vi "Lockin.DAQ.Generate.Waveforms.vi"(4 "sweep index":i32=-1, 6 "Reset Phase?":bool, 8 "error in (no error)":errorcluster, 11 "Instrument.DAQ":refnum<class "Instrument.DAQ.lvclass">) -> (0 "error out":errorcluster, 3 "Instrument.DAQ":refnum<class "Instrument.DAQ.lvclass">)   [LabVIEW 2019, in "Instrument.DAQ.lvclass"]
uses:
  Instrument.DAQ.lvclass
  Instrument.DAQ.lvclass/Instrument.DAQ.ctl
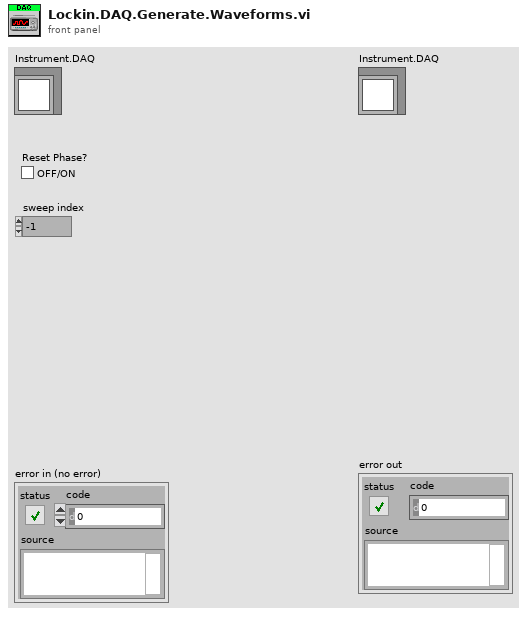
[diagram p1: front panel]
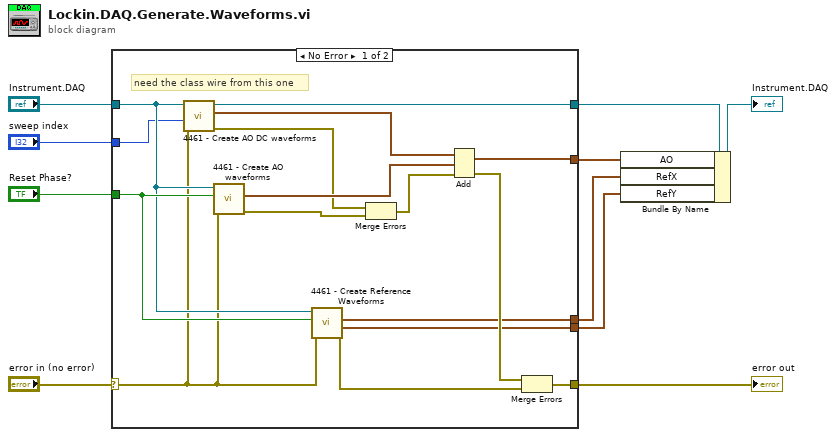
[diagram p0: block diagram]
diagram:
  n1 = case shown="No Error" "error in (no error)" {
    selector: "error in (no error)" -> [w23 w28]
    tunnel: [w11 _] -> w2
    tunnel: "Reset Phase?" -> [w26 _]
    tunnel: [w18 _] -> w3
    tunnel: [w25 w28] -> w9
    tunnel: "Instrument.DAQ" -> [w24 w27]
    tunnel: "sweep index" -> [w12 _]
    tunnel: [w19 w27] -> w4
    tunnel: [w13 _] -> w1
    frame No Error {
      # "need the class wire from this one"
      n2 = call "4461 - Create AO DC waveforms.vi"("error in (no error)"=w23, "sweep index"=w12, "Instrument.DAQ in"=w24) -> ("error out"=w14:errorcluster, "AO Array"=w17:waveform(dbl)[], "Instrument.DAQ out"=w19:refnum<class "Instrument.DAQ.lvclass">)  [unwired: 6 in]
      n3 = call "4461 - Create AO waveforms.vi"("error in (no error)"=w23, "reset phase"=w26, "Lockin.DAQ"=w24) -> ("error out"=w15:errorcluster, "AO Array"=w16:waveform(dbl)[])  [unwired: 6 in, 1 out]
      n4 = call "4461 - Create Reference Waveforms.vi"("error in (no error)"=w23, "reset phase"=w26, "Lockin.DAQ in"=w24) -> ("error out"=w22:errorcluster, "Y"=w13:waveform(dbl)[], "X"=w11:waveform(dbl)[])  [unwired: 5 in, 1 out]
      n5 = Merge Errors(w14, w15) -> (w20:errorcluster)
      n6 = Add(1:w16, 2:w17, 4:w20) -> (0:w18:waveform(dbl)[], 3:w21:errorcluster)
      n7 = Merge Errors(w21, w22) -> (w25:errorcluster)
    }
    frame Error {
    }
  }
  "error out" <- w9
  n8 = Bundle By Name(cluster=w4, "AO"=w3, "RefX"=w2, "RefY"=w1) -> (→"Instrument.DAQ":refnum<class "Instrument.DAQ.lvclass">)
